vi "释放通道后申请通道_RF.vi"(8 "error in":errorcluster) -> (0 "error out":errorcluster)   [LabVIEW 2015]
uses:
  Global/SeverGlobal.vi
panel:
  out "ack":string
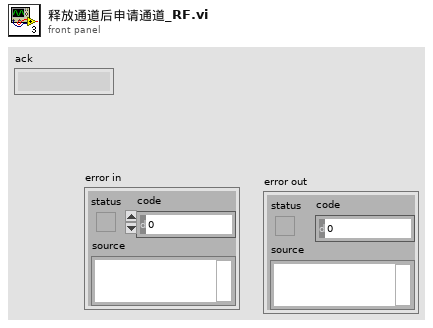
[diagram p1: front panel]
types:
  T1 = enum16{"open", "replace", "create", "open or create", "replace or create", "replace or create with confirmation"}
  T2 = typedef "响应消息头.ctl" = string
  T3 = cluster{"TCP Ref":refnum<k5>, "IP":string, "userName":string, "A":u16, "COM":u16, "time":u32}[]
  T4 = typedef "队列.ctl" = cluster{"COM1":refnum<queue>, "COM2":refnum<queue>, "COM3":refnum<queue>, "COM4":refnum<queue>, "OUT1":refnum<queue>, "OUT2":refnum<queue>, "OUT3":refnum<queue>, "OUT4":refnum<queue>, "OUT5":refnum<queue>, "OUT6":refnum<queue>, "OUT7":refnum<queue>, "OUT8":refnum<queue>}
  T5 = cluster{"TCP Ref":refnum<k5>, "Broadcast":refnum<k5>, "TF Ref":refnum<k5>, "IP":string, "port":u16, "userName":string, "passWord":string, "authority":string}[]
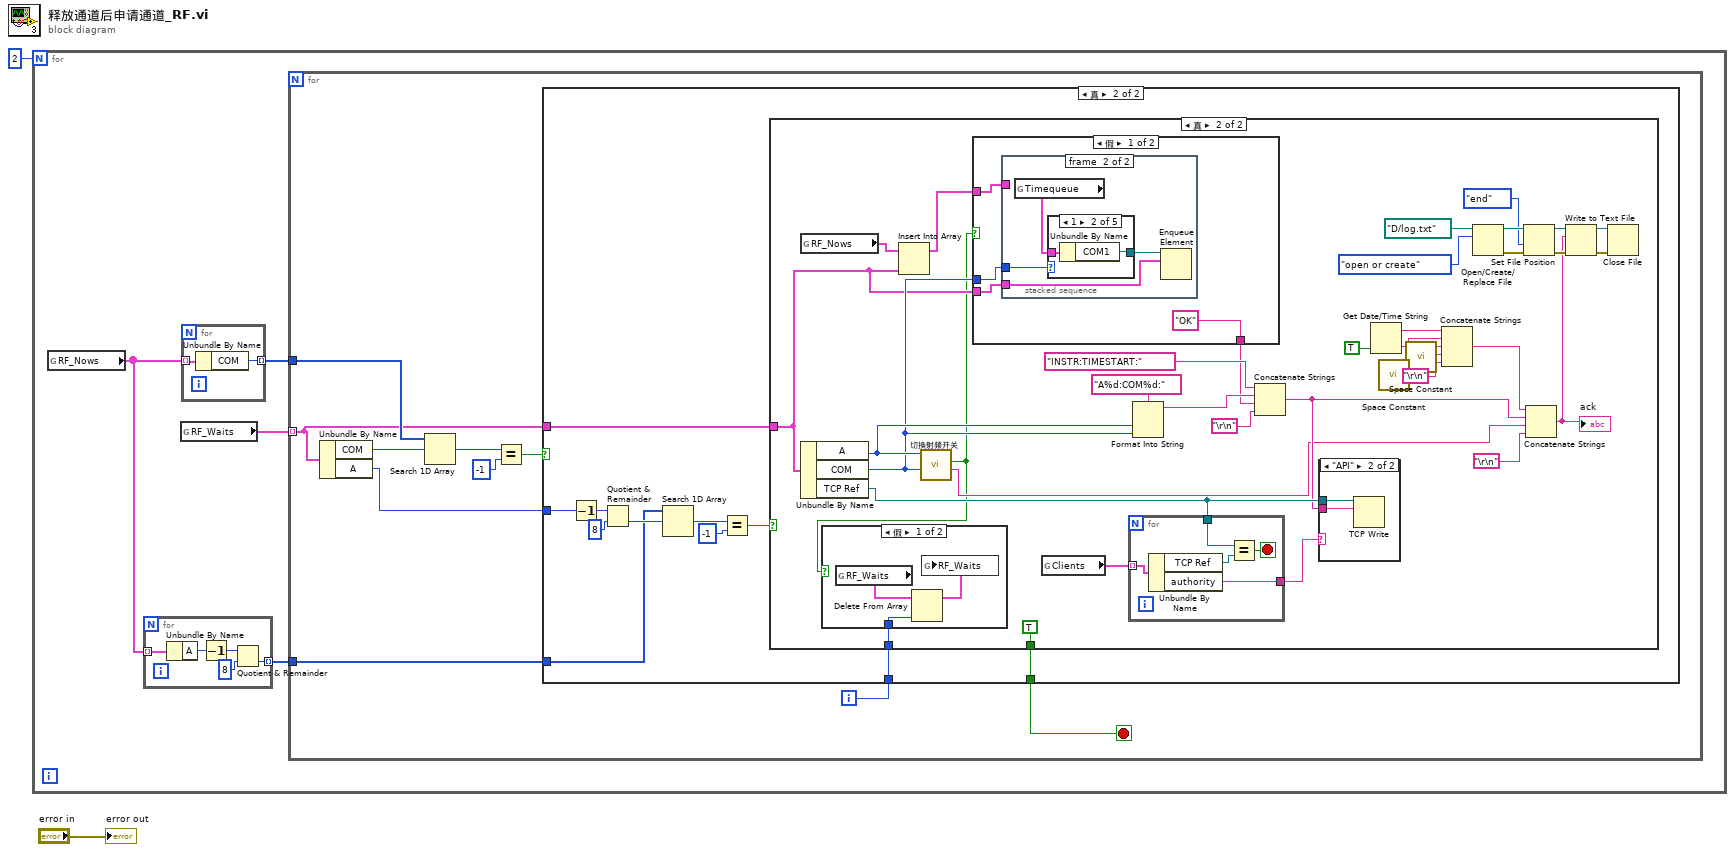
[diagram p0: block diagram]
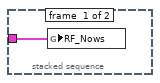
[diagram p5: hidden frame]
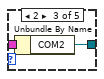
[diagram p7: hidden frame]
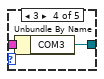
[diagram p8: hidden frame]
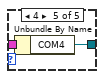
[diagram p9: hidden frame]
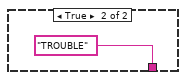
[diagram p10: hidden frame]
diagram:
  n1 = for {
    N: 2 -> [_]
    n2 = global read "SeverGlobal.vi" "RF_Nows"() -> (w4:T3)
    n3 = for {
      tunnel: w4 -> [w11] mode=indexing
      tunnel: [w7] -> w3 mode=indexing
      n4 = Unbundle By Name(w11) -> ("A"=w8:u16)
      n5 = Decrement(x=w8) -> (x-1=w9:u16)
      n6 = Quotient & Remainder(x=w9, y=8) -> (floor(x/y)=w7:i32)  [unwired: 1 out]
    }
    n7 = global read "SeverGlobal.vi" "RF_Waits"() -> (w6:T3)
    n8 = for {
      tunnel: w4 -> [w98] mode=indexing
      tunnel: [w97] -> w5 mode=indexing
      n9 = Unbundle By Name(w98) -> ("COM"=w97:u16)
    }
    n10 = for {
      tunnel: w6 -> [w14] mode=indexing
      tunnel: w5 -> [w18]
      tunnel: w3 -> [w16]
      i -> [w12]
      stop <- w13 stop-if-true
      n11 = Unbundle By Name(w14) -> ("COM"=w19:u16, "A"=w15:u16)
      n12 = Search 1D Array(1D array=w18, element=w19) -> (index of element=w21:i32)  [unwired: 1 in]
      n13 = Equal?(x=w21, y=-1) -> (x = y?=w17:bool)
      n14 = case shown="真" w17 {
        tunnel: w16 -> [_ w27]
        tunnel: w15 -> [_ w26]
        tunnel: w14 -> [_ w24]
        tunnel: [_ w23] -> w13
        tunnel: w12 -> [_ w22]
        frame False {
          # "COM冲突，不作为"
        }
        frame True {
          n15 = Decrement(x=w26) -> (x-1=w28:u16)
          n16 = Quotient & Remainder(x=w28, y=8) -> (floor(x/y)=w32:i32)  [unwired: 1 out]
          n17 = Search 1D Array(1D array=w27, element=w32) -> (index of element=w30:i32)  [unwired: 1 in]
          n18 = Equal?(x=w30, y=-1) -> (x = y?=w25:bool)
          n19 = case shown="真" w25 {
            tunnel: w24 -> [_ w55]
            tunnel: [_ TRUE] -> w23
            tunnel: w22 -> [_ w66]
            frame False {
              # "A冲突，不作为"
            }
            frame True {
              n20 = global read "SeverGlobal.vi" "RF_Nows"() -> (w68:T3)
              n21 = Unbundle By Name(w55) -> ("A"=w61:u16, "COM"=w56:u16, "TCP Ref"=w59:refnum<k5>)
              n22 = Insert Into Array(array=w68, new element=w55) -> (w57:T3)  [unwired: 1 in]
              n23 = call "切换射频开关.vi"("COM"=w56, "A"=w61) -> ("ask"=w36:string, "Isfailed"=w33:bool)  [unwired: 7 in, 1 out]
              n24 = case shown="假" w33 {
                tunnel: w66 -> [w70 _]
                frame False {
                  n25 = global read "SeverGlobal.vi" "RF_Waits"() -> (w71:T3)
                  n26 = Delete From Array(array=w71, index=w70) -> (array with subset deleted=w69:T3)  [unwired: 1 in, 1 out]
                  n27 = global write "SeverGlobal.vi" "RF_Waits"(w69) -> ()
                }
                frame True {
                }
              }
              n28 = case shown="假" w33 {
                tunnel: w57 -> [w75 _]
                tunnel: w56 -> [w74 _]
                tunnel: w55 -> [w73 _]
                tunnel: ["OK" ("format string") "TROUBLE" ("format string")] -> w34
                frame False {
                  n29 = stacked-sequence {
                    tunnel: w75 -> [w76 _]
                    tunnel: w74 -> [_ w78]
                    tunnel: w73 -> [_ w77]
                    frame #0 {
                      n30 = global write "SeverGlobal.vi" "RF_Nows"(w76) -> ()
                    }
                    frame #1 {
                      n31 = global read "SeverGlobal.vi" "Timequeue"() -> (w80:T4)
                      n32 = case shown="1" w78 {
                        tunnel: w80 -> [_ w82 w84 w86 w88]
                        tunnel: [_ w81 w83 w85 w87] -> w79
                        frame 0, Default {
                        }
                        frame 1 {
                          n33 = Unbundle By Name(w82) -> ("COM1"=w81:refnum<queue>)
                        }
                        frame 2 {
                          n34 = Unbundle By Name(w84) -> ("COM2"=w83:refnum<queue>)
                        }
                        frame 3 {
                          n35 = Unbundle By Name(w86) -> ("COM3"=w85:refnum<queue>)
                        }
                        frame 4 {
                          n36 = Unbundle By Name(w88) -> ("COM4"=w87:refnum<queue>)
                        }
                      }
                      n37 = Enqueue Element(queue=w79, element=w77) -> ()  [unwired: 2 in, 3 out]
                    }
                  }
                }
                frame True {
                }
              }
              n38 = global read "SeverGlobal.vi" "Clients"() -> (w60:T5)
              n39 = for {
                tunnel: w60 -> [w96] mode=indexing
                tunnel: w59 -> [w94]
                tunnel: [w92] -> w58
                stop <- w93 stop-if-true
                n40 = Unbundle By Name(w96) -> ("TCP Ref"=w95:refnum<k5>, "authority"=w92:string)
                n41 = Equal?(x=w94, y=w95) -> (x = y?=w93:bool)
              }
              n42 = Format Into String(format string="A%d:COM%d:", w61, w56) -> (resulting string=w63:string)  [unwired: 2 in, 1 out]
              n43 = Concatenate Strings(T2 "INSTR:TIMESTART:" ("Combo Box"), w63, w34, "\r\n") -> (w47:string)
              n44 = case shown="\"API\"" w58 {
                tunnel: w47 -> [_ w91]
                tunnel: w59 -> [_ w90]
                frame Default {
                }
                frame "API" {
                  n45 = TCP Write(connection ID=w90, data in=w91) -> ()  [unwired: 2 in, 3 out]
                }
              }
              n46 = Get Date/Time String(want seconds? (F)=TRUE ("需要秒？(F)")) -> (date string=w53:string, time string=w52:string)  [unwired: 2 in]
              n47 = call <vilib>:"Space Constant.vi"() -> ("String"=w51:string)
              n48 = call <vilib>:"Space Constant.vi"() -> ("String"=w50:string)
              n49 = Concatenate Strings(w53, w51, w52, w50, "\r\n") -> (w48:string)
              n50 = Open/Create/Replace File(file path (use dialog)=path "D:/log.txt" ("文件（使用对话框）"), operation (0:open)=T1."open or create" ("操作(0:open)")) -> (refnum out=w43:refnum<file>, error out=w44:errorcluster)  [unwired: 4 in, 1 out]
              n51 = Set File Position(refnum=w43, from (0:start)=enum16{"start", "end", "current"}."end" ("自（0:起始）"), error in=w44) -> (refnum out=w45:refnum<file>, error out=w46:errorcluster)  [unwired: 1 in]
              n52 = Concatenate Strings(w48, w47, w36, "\r\n") -> (w37:string)
              "ack" <- w37
              n53 = Write to Text File(file (use dialog)=w45, text=w37, error in=w46) -> (refnum out=w41:refnum<file>, error out=w40:errorcluster)  [unwired: 1 in, 1 out]
              n54 = Close File(refnum=w41, error in=w40) -> ()  [unwired: 2 out]
            }
          }
        }
      }
    }
  }
  "error out" <- "error in"
